vi "Read All Control Values.vi"(8 "error in (no error)":errorcluster, 11 "CD Parameter Manager in":refnum<class "CD Parameter Manager.lvclass">) -> (0 "error out":errorcluster, 3 "CD Parameter Manager out":refnum<class "CD Parameter Manager.lvclass">)   [LabVIEW 2016, in "CD Parameter Manager API.lvlib" / "CD Parameter Manager.lvclass"]
uses:
  CD Parameter Manager.lvclass
  Parameter Class/Parameter.lvclass
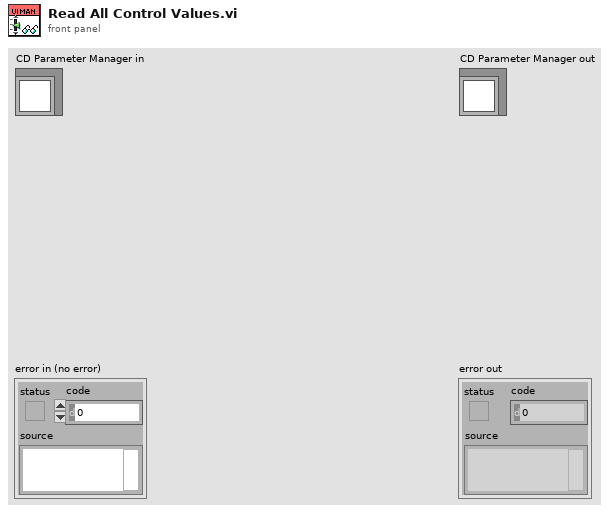
[diagram p1: front panel]
types:
  T1 = cluster{"Group name":string, "Controls":refnum<class "Parameter.lvclass">[]}[]
  T2 = cluster{"Group name":string, "Controls":refnum<class "Parameter.lvclass">[]}
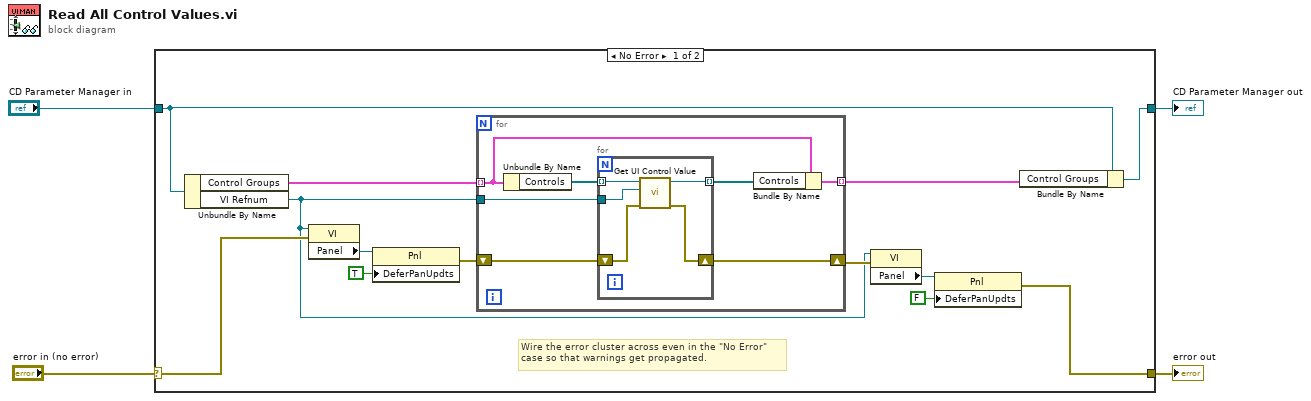
[diagram p0: block diagram]
diagram:
  n1 = case shown="No Error" "error in (no error)" {
    selector: "error in (no error)" -> [w12 w31]
    tunnel: [w6 w31] -> w3
    tunnel: [w15 w30] -> w1
    tunnel: "CD Parameter Manager in" -> [w16 w30]
    frame No Error {
      # "Wire the error cluster across even in the \"No Error\"\ncase so that warnings get propagated."
      n2 = Unbundle By Name(w16) -> ("Control Groups"=w17:T1, "VI Refnum"=w5:refnum<vi>)
      n3 = property class="VI"(reference=w5, error in=w12) -> ("Panel"=w13:refnum<vi>)  [unwired: 2 out]
      n4 = property class="Pnl"(reference=w13, "DeferPanUpdts"=TRUE ("Defer Panel Updates")) -> (error out=w11:errorcluster)  [unwired: 1 in, 1 out]
      n5 = for {
        tunnel: w5 -> [w24]
        tunnel: w17 -> [w19] mode=indexing
        shift-right: [w22] -> w7
        shift-left: w11 -> [w23]
        tunnel: [w18] -> w14 mode=indexing
        n6 = Unbundle By Name(w19) -> ("Controls"=w21:refnum<class "Parameter.lvclass">[])
        n7 = for {
          tunnel: w24 -> [w29]
          tunnel: w21 -> [w28] mode=indexing
          shift-right: [w26] -> w22
          shift-left: w23 -> [w27]
          tunnel: [w25] -> w20 mode=indexing
          n8 = call-dynamic "Get UI Control Value.vi"("error in (no error)"=w27, "VI Ref"=w29, "Parameter in"=w28) -> ("error out"=w26:errorcluster, "Parameter out"=w25:refnum<class "Parameter.lvclass">)  [unwired: 7 in]
        }
        n9 = Bundle By Name(cluster=w19, "Controls"=w20) -> (w18:T2)
      }
      n10 = property class="VI"(reference=w5, error in=w7) -> ("Panel"=w8:refnum<vi>)  [unwired: 2 out]
      n11 = property class="Pnl"(reference=w8, "DeferPanUpdts"=FALSE ("Defer Panel Updates")) -> (error out=w6:errorcluster)  [unwired: 1 in, 1 out]
      n12 = Bundle By Name(cluster=w16, "Control Groups"=w14) -> (w15:refnum<class "CD Parameter Manager.lvclass">)
    }
    frame Error {
    }
  }
  "error out" <- w3
  "CD Parameter Manager out" <- w1
